vi "CheckPythonExtension.vi"(11 "path in":path) -> (3 "path out":path)   [LabVIEW 2020]
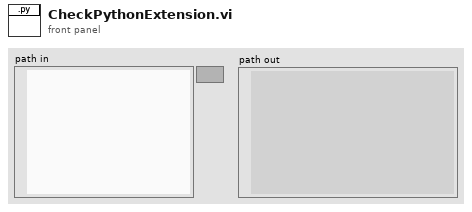
[diagram p1: front panel]
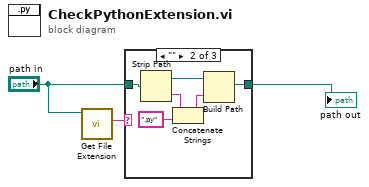
[diagram p0: block diagram]
diagram:
  n1 = call <vilib>:"Get File Extension.vi"("file"="path in") -> ("lowercase file extension"=w1:string)  [unwired: 6 in, 4 out]
  n2 = case shown="\"\"" w1 {
    tunnel: [w4 w9 w11] -> w2
    tunnel: "path in" -> [w4 w10 w11]
    frame Default {
    }
    frame "" {
      n3 = Strip Path(path=w10) -> (stripped path=w6:path, name=w8:string)
      n4 = Concatenate Strings(w8, ".py" ("string")) -> (w7:string)
      n5 = Build Path(base path=w6, name or relative path=w7) -> (appended path=w9:path)
    }
    frame "py" {
    }
  }
  "path out" <- w2
